vi "Change Container Lease ID.vi"(4 "Proposed Lease ID":string, 6 "Current Lease ID":string, 8 "error in (no error)":errorcluster, 10 "Container":string, 11 "Azure Session in":refnum<class "Session.lvclass">) -> (0 "error out":errorcluster, 3 "Azure Session out":refnum<class "Session.lvclass">)   [LabVIEW 2015, in "NI_Azure_Blob.lvlib"]
doc: "Change the ID of an existing lease on a container."
uses:
  NI_Azure_Blob.lvlib
  Core/Session/Session.lvclass
  Core/Name Value Pair.ctl
  Lease Action.ctl
  Core/Session/Session.lvclass/Session.ctl
  Core/Session/Write Request Headers.vi
  Core/Session/Write Request Parameters.vi
  Core/Session/Write HTTP Verb.vi
  Core/Session/Write URL Suffix.vi
  Core/NI_Azure_Core.lvlib
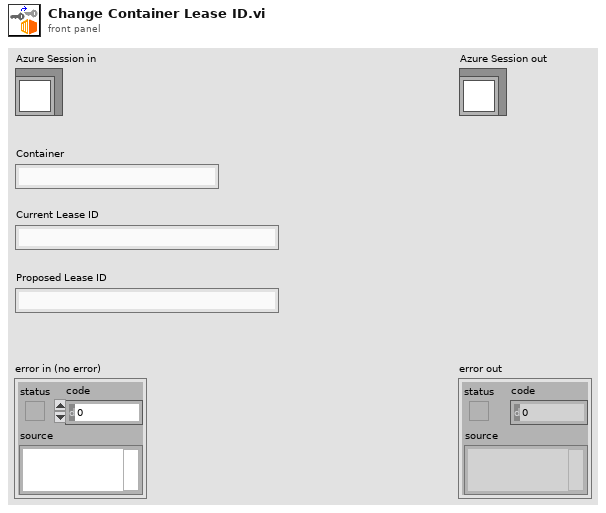
[diagram p1: front panel]
types:
  T1 = typedef "NI_Azure_Blob.lvlib/Lease Action.ctl" = enum16{"acquire", "renew", "change", "release", "break"}
  T2 = typedef "NI_Azure_Core.lvlib/Name Value Pair.ctl" = cluster{"name":string, "value":string}
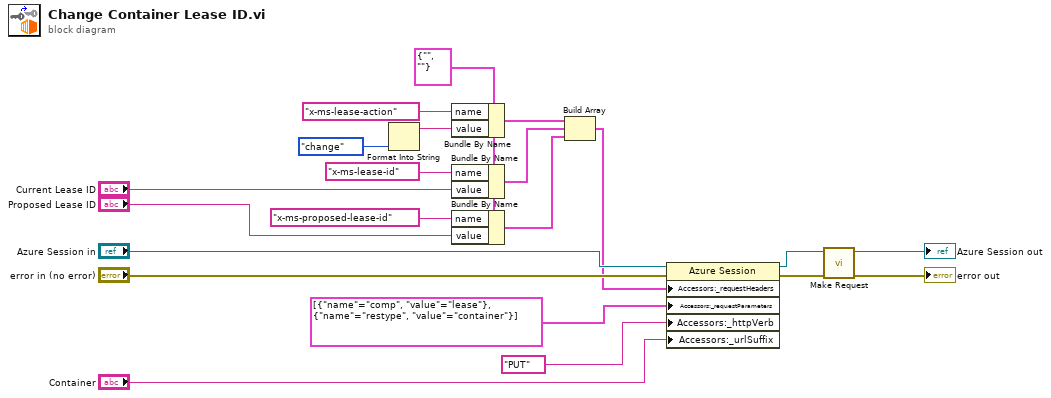
[diagram p0: block diagram]
diagram:
  w10 = T2 {"name"="", "value"=""} ("Cluster")
  n1 = Format Into String(Lease_Action."change" ("Lease action")) -> (resulting string=w15:string)  [unwired: 3 in, 1 out]
  n2 = Bundle By Name(cluster=w10, "name"="x-ms-lease-action" ("header"), "value"=w15) -> (w17:T2)
  n3 = Bundle By Name(cluster=w10, "name"="x-ms-lease-id" ("header"), "value"="Current Lease ID") -> (w11:T2)
  n4 = Bundle By Name(cluster=w10, "name"="x-ms-proposed-lease-id" ("header"), "value"="Proposed Lease ID") -> (w9:T2)
  n5 = Build Array(w17, w11, w9) -> (w4:T2[])
  n6 = property class="Azure Session"(reference="Azure Session in", error in="error in (no error)", "Accessors:_requestHeaders"=w4, "Accessors:_requestParameters"=T2[] [{"name"="comp", "value"="lease"}, {"name"="restype", "value"="container"}] ("request parameters"), "Accessors:_httpVerb"="PUT" ("HTTP-Verb"), "Accessors:_urlSuffix"="Container") -> (reference out=w5:refnum<class "Session.lvclass">, error out=w7:errorcluster)
  n7 = call "Make Request.vi"("error in (no error)"=w7, "Session in"=w5) -> ("error out"=→"error out":errorcluster, "Session out"=→"Azure Session out":refnum<class "Session.lvclass">)  [unwired: 7 in, 1 out]
